vi "Realsense Cam Frame Get.vi"(8 "error in (no error)":errorcluster, 11 "Realsense Cam in":refnum<class "Realsense Cam.lvclass">) -> (0 "error out":errorcluster, 3 "Realsense Cam out":refnum<class "Realsense Cam.lvclass">)   [LabVIEW 2018, in "Realsense Cam.lvclass"]
uses:
  Realsense Cam.lvclass
  Realsense Cam.lvclass/Realsense Cam.ctl
  realsense_wrapper_api/libRealSense3.lvlib
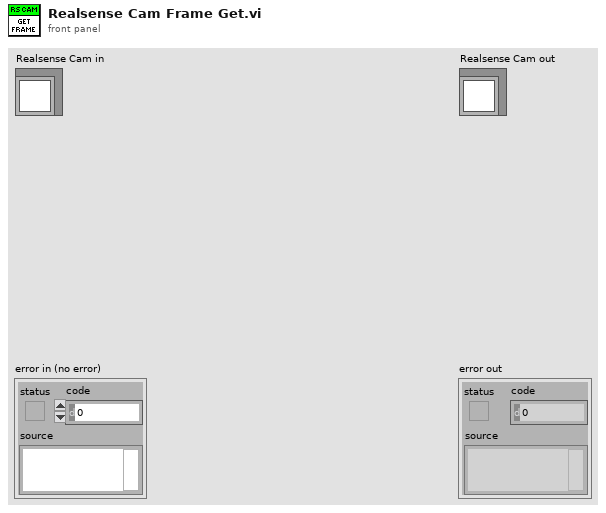
[diagram p1: front panel]
types:
  T1 = cluster{"Subsample":bool, "Spatial filter":bool, "Temporal filter":bool}
  T2 = cluster{"decimation filter block":u64, "spatial filter block":u64, "temporal filter block":u64, "disparity_transforg_2_block":u64, "disparity_transforg_1_block":u64}
  T3 = cluster{"decimation filter queue":u64, "spatial filter queue":u64, "temporal filter queue":u64, "disparity_transforg_2_queue":u64, "disparity_transforg_1_queue":u64}
  T4 = cluster{"Decimation Scale (1-10)":u8, "Spatial Alpha\n(0-1)":sgl, "Spatial Delta \n(1/32 disp)":u16, "Temporal Alpha\n(0-1)":sgl, "Temporal Delta\n(1/32 disp)":u16, "Persistence (0= none, 8=max)":u8, "spatial holefill radius\n(0 disable, 5 max) ":u8, "spatial iteration\n(2=default)":u8}
  T5 = enum16{"Depth", "Color (ext.)", "Color (left) ", "IR Left", "IR Right", "IR Left (Y16)", "IR Right (Y16)"}
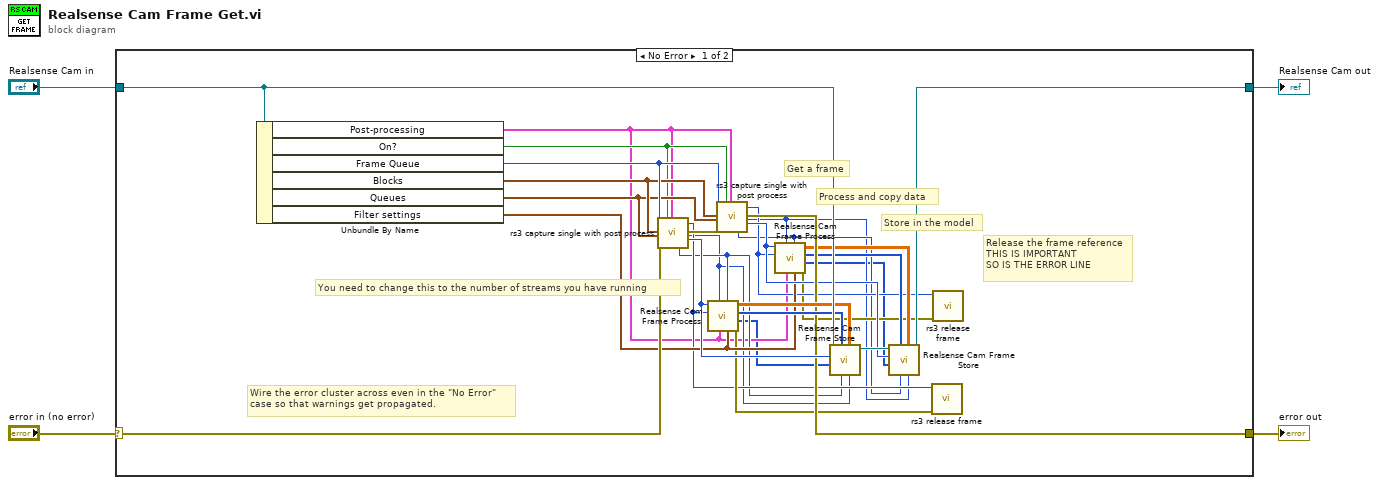
[diagram p0: block diagram]
diagram:
  n1 = case shown="No Error" "error in (no error)" {
    selector: "error in (no error)" -> [w27 w34]
    tunnel: [w21 w34] -> w3
    tunnel: [w17 w33] -> w1
    tunnel: "Realsense Cam in" -> [w26 w33]
    frame No Error {
      # "Release the frame reference\nTHIS IS IMPORTANT\nSO IS THE ERROR LINE"
      # "Store in the model"
      # "Process and copy data"
      # "Get a frame"
      # "You need to change this to the number of streams you have running"
      # "Wire the error cluster across even in the \"No Error\"\ncase so that warnings get propagated."
      n2 = Unbundle By Name(w26) -> ("Post-processing"=w7:T1, "On?"=w28:bool, "Frame Queue"=w31:u64, "Blocks"=w30:T2, "Queues"=w29:T3, "Filter settings"=w16:T4)
      n3 = call "rs3 capture single with post process.vi"("frame queue in"=w31, "Processing Blocks"=w30, "Processing Queues"=w29, "error in (no error)"=w27, "PostProcess"=w28, "Post-processing"=w7) -> ("height"=w11:i32, "Processed frame out"=w14:u64, "error out"=w32:errorcluster, "width"=w10:i32, "Stream type"=w23:T5)  [unwired: 8 in, 9 out]
      n4 = call "Realsense Cam Frame Process.vi"("Filter settings"=w16, "Height"=w11, "Settings"=w7, "Width"=w10, "Frame Data"=w14, "Stream type"=w23) -> ("error out"=w15:errorcluster, "16-Bit Data"=w6:u16[], "Bytes"=w24:u8[], "Depth"=w25:sgl[][])  [unwired: 2 in]
      n5 = call "rs3 capture single with post process.vi"("frame queue in"=w31, "Processing Blocks"=w30, "Processing Queues"=w29, "error in (no error)"=w32, "PostProcess"=w28, "Post-processing"=w7) -> ("height"=w9:i32, "Processed frame out"=w13:u64, "error out"=w21:errorcluster, "width"=w8:i32, "Stream type"=w18:T5)  [unwired: 8 in, 9 out]
      n6 = call "Realsense Cam Frame Process.vi"("Filter settings"=w16, "Height"=w9, "Settings"=w7, "Width"=w8, "Frame Data"=w13, "Stream type"=w18) -> ("error out"=w12:errorcluster, "16-Bit Data"=w5:u16[], "Bytes"=w19:u8[], "Depth"=w20:sgl[][])  [unwired: 2 in]
      n7 = call-dynamic "Realsense Cam Frame Store.vi"("Width"=w10, "Depths"=w25, "Height"=w11, "Bytes"=w24, "16-Bit IR"=w6, "Stream type"=w23, "Realsense Cam in"=w26) -> ("Realsense Cam out"=w22:refnum<class "Realsense Cam.lvclass">)  [unwired: 3 in, 1 out]
      n8 = call-dynamic "Realsense Cam Frame Store.vi"("Width"=w8, "Depths"=w20, "Height"=w9, "Bytes"=w19, "16-Bit IR"=w5, "Stream type"=w18, "Realsense Cam in"=w22) -> ("Realsense Cam out"=w17:refnum<class "Realsense Cam.lvclass">)  [unwired: 3 in, 1 out]
      n9 = call "rs3 release frame.vi"("error in (no error)"=w15, "Frame"=w14) -> ()  [unwired: 8 in, 2 out]
      n10 = call "rs3 release frame.vi"("error in (no error)"=w12, "Frame"=w13) -> ()  [unwired: 8 in, 2 out]
    }
    frame Error {
    }
  }
  "error out" <- w3
  "Realsense Cam out" <- w1
